vi "Copy LogFile to Location.vi"(5 "Local Save path":path, 7 "System Definition Path":path, 8 "error in (no error)":errorcluster, 11 "Target Refnum in":refnum<k24>) -> (0 "error out":errorcluster, 2 "File Succesfuly copied":bool, 3 "Target Refnum out":refnum<k24>)   [LabVIEW 2019, in "TLCD System Tests.lvclass"]
uses:
  TLCD System Tests.lvclass
  NationalInstruments.VeriStand.SystemDefinitionAPI
  <vilib>/WebDAVClient/Advanced/Get File.vi
  TLCD Test Class/TLCD Test Class.lvclass
  <vilib>/WebDAVClient/NI_WebDAV.lvlib
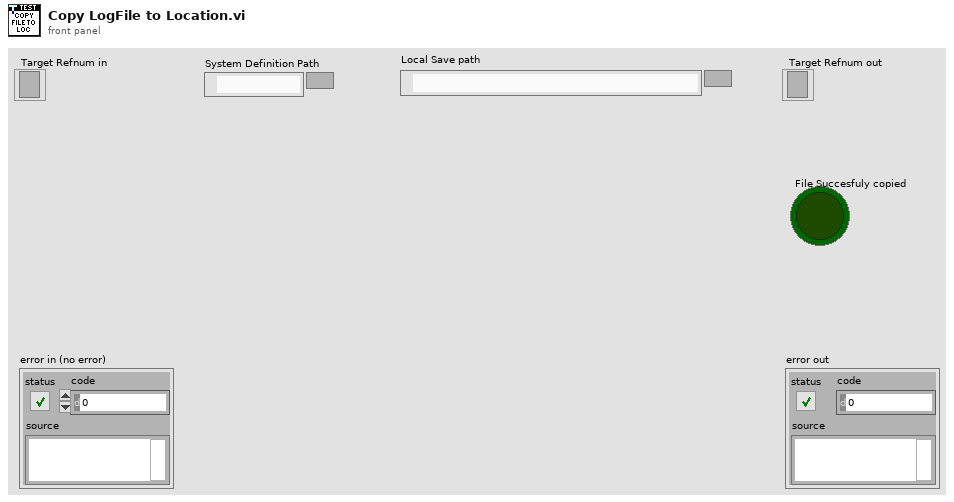
[diagram p1: front panel]
types:
  T1 = typedef "NI_WebDAV.lvlib/SessionHandle.ctl" = refnum<k1>
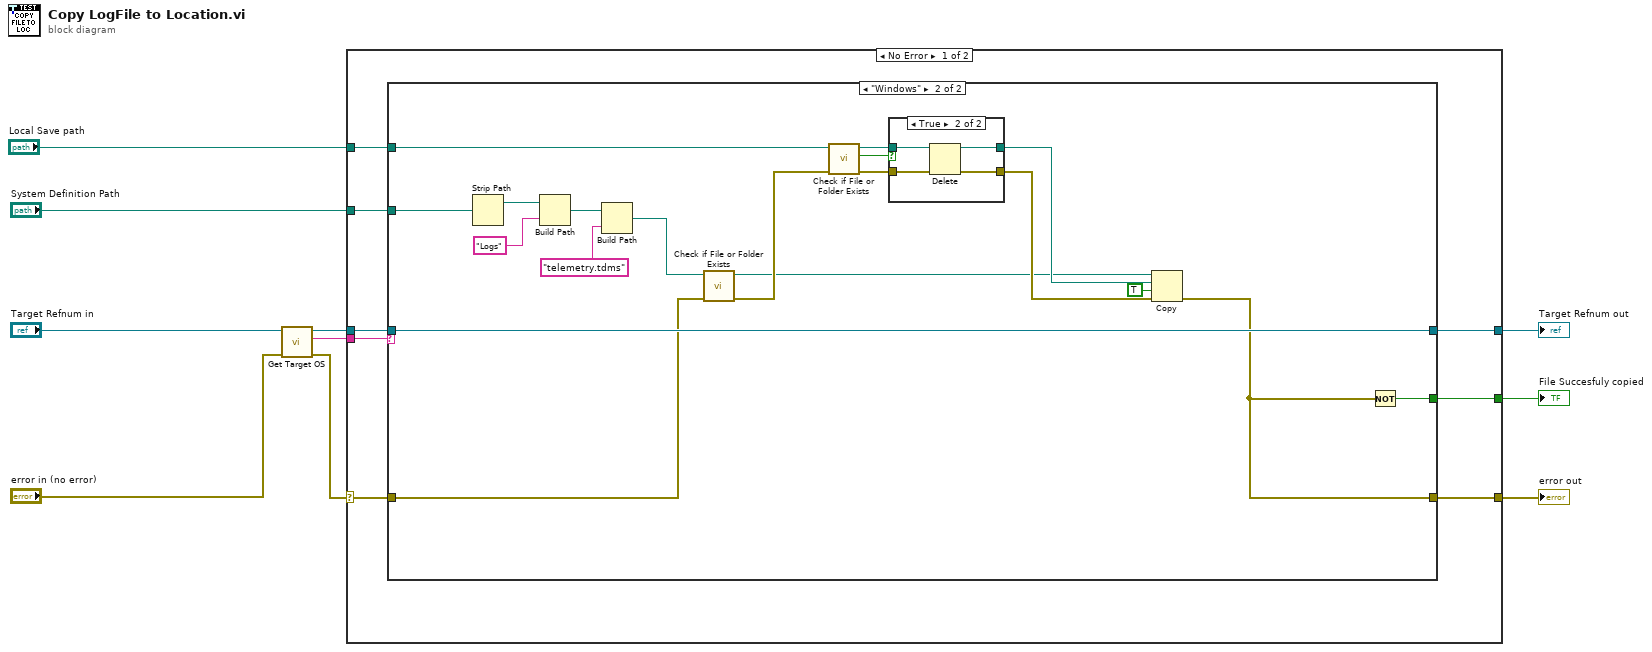
[diagram p0: block diagram]
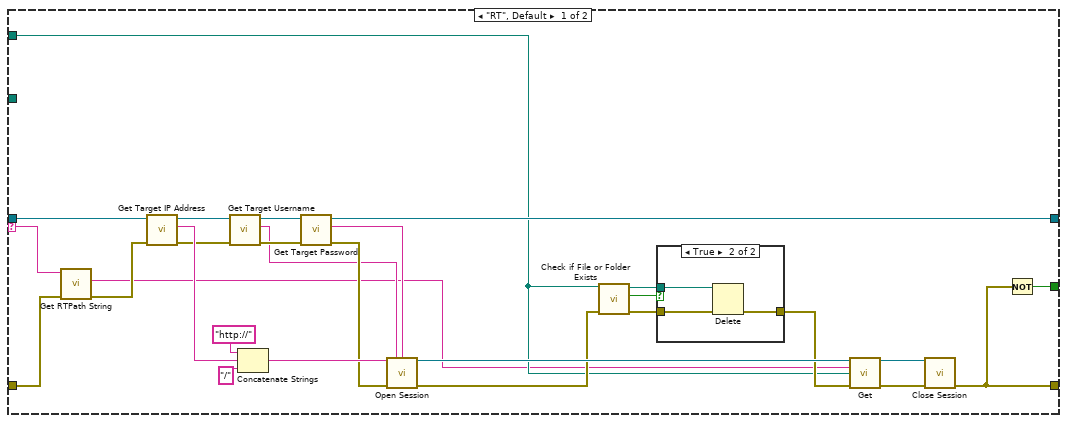
[diagram p2: hidden frame]
diagram:
  n1 = call "Get Target OS.vi"("error in (no error)"="error in (no error)", "Target ref in"="Target Refnum in") -> ("error out"=w3:errorcluster, "OperatingSystem"=w9:string, "Target ref out"=w8:refnum<k24>)  [unwired: 7 in]
  n2 = case shown="No Error" w3 {
    selector: w3 -> [w13 w77]
    tunnel: "System Definition Path" -> [w18 _]
    tunnel: w9 -> [w17 _]
    tunnel: w8 -> [w16 w76]
    tunnel: [w15 w76] -> w5
    tunnel: [w14 w77] -> w4
    tunnel: "Local Save path" -> [w12 _]
    tunnel: [w11 _] -> w1
    frame No Error {
      n3 = case shown="\"Windows\"" w17 {
        selector: w17 -> [w46 _]
        tunnel: [w20 w52] -> w14
        tunnel: [w31 w69] -> w15
        tunnel: w13 -> [w45 w62]
        tunnel: w16 -> [w44 w69]
        tunnel: w18 -> [_ w68]
        tunnel: w12 -> [w22 w58]
        tunnel: [w19 w51] -> w11
        frame "RT", Default {
          n4 = call "Get RTPath String.vi"("error in (no error)"=w45, "Target OS in"=w46) -> ("error out"=w43:errorcluster, "RT File Path"=w21:string)  [unwired: 6 in, 2 out]
          n5 = call "Get Target IP Address.vi"("error in (no error)"=w43, "Target ref in"=w44) -> ("error out"=w36:errorcluster, "IPAddress"=w41:string, "Target ref out"=w38:refnum<k24>)  [unwired: 7 in]
          n6 = call "Get Target Username.vi"("error in (no error)"=w36, "Target ref in"=w38) -> ("error out"=w35:errorcluster, "Username"=w32:string, "Target ref out"=w37:refnum<k24>)  [unwired: 7 in]
          n7 = Concatenate Strings("http://" ("string"), w41, "/" ("string")) -> (w39:string)
          n8 = call "Get Target Password.vi"("error in (no error)"=w35, "Target ref in"=w37) -> ("error out"=w34:errorcluster, "Password"=w33:string, "Target ref out"=w31:refnum<k24>)  [unwired: 7 in]
          n9 = call <vilib>:"Open Session.vi"("host uri prefix"=w39, "username"=w32, "password"=w33, "error in (no error)"=w34) -> ("session handle out"=w30:T1, "error out"=w27:errorcluster)  [unwired: 10 in]
          n10 = call <vilib>:"Check if File or Folder Exists.vi"("error in (no error)"=w27, "path"=w22) -> ("error out"=w23:errorcluster, "file or folder exists?"=w25:bool, "dup path"=w24:path)  [unwired: 7 in]
          n11 = case shown="True" w25 {
            tunnel: w24 -> [_ w50]
            tunnel: w23 -> [w47 w49]
            tunnel: [w47 w48] -> w26
            frame False {
            }
            frame True {
              n12 = Delete(path (use dialog)=w50, error in=w49) -> (error out=w48:errorcluster)  [unwired: 3 in, 2 out]
            }
          }
          n13 = call-poly <vilib>:"Get.vi"("session handle"=w30, "relative uri"=w21, "local file path"=w22, "error in (no error)"=w26) -> ("session handle out"=w29:T1, "error out"=w28:errorcluster)  [unwired: 9 in, 1 out]
          n14 = call <vilib>:"Close Session.vi"("session handle"=w29, "error in (no error)"=w28) -> ("error out"=w20:errorcluster)  [unwired: 13 in]
          n15 = Not(x=w20) -> (.not. x?=w19:bool)
        }
        frame "Windows" {
          n16 = Strip Path(path=w68) -> (stripped path=w67:path)  [unwired: 1 out]
          n17 = Build Path(base path=w67, name or relative path="Logs") -> (appended path=w65:path)
          n18 = Build Path(base path=w65, name or relative path="telemetry.tdms") -> (appended path=w63:path)
          n19 = call <vilib>:"Check if File or Folder Exists.vi"("error in (no error)"=w62, "path"=w63) -> ("error out"=w57:errorcluster, "dup path"=w54:path)  [unwired: 7 in, 1 out]
          n20 = call <vilib>:"Check if File or Folder Exists.vi"("error in (no error)"=w57, "path"=w58) -> ("error out"=w59:errorcluster, "file or folder exists?"=w61:bool, "dup path"=w60:path)  [unwired: 7 in]
          n21 = case shown="True" w61 {
            tunnel: w60 -> [w70 w75]
            tunnel: w59 -> [w71 w74]
            tunnel: [w71 w73] -> w56
            tunnel: [w70 w72] -> w55
            frame False {
            }
            frame True {
              n22 = Delete(path (use dialog)=w75, error in=w74) -> (deleted path=w72:path, error out=w73:errorcluster)  [unwired: 3 in, 1 out]
            }
          }
          n23 = Copy(8:w56, 9:TRUE ("overwrite (F)"), 10:w55, 11:w54) -> (0:w52:errorcluster)  [unwired: 1 in, 2 out]
          n24 = Not(x=w52) -> (.not. x?=w51:bool)
        }
      }
    }
    frame Error {
    }
  }
  "Target Refnum out" <- w5
  "error out" <- w4
  "File Succesfuly copied" <- w1
